vi "ROI entry-bundle parameter values.vi"(7 "XYZ_Coordinates":T1[](array[typedef]) {"Apparent Frame Size" format="%#_6f"; "Original FOV (um)" format="%#_6f"; "Pixels per miniscan" format="%#_6f"; "Dwell Time per pixel" format="%#_6f"; "Resolution" format="%#_6f"; "ROI group ID" format="%#_6f"; "Laser Power (%)" format="%#_6f"; "Zoom" format="%#_6f"; "Frame Size" format="%#_6f"; "Number of lines" format="%#_6f"; "Composite ID" format="%#_6f"; "Angle (deg)" format="%#_6f"; "ROI Time (ns)" format="%#_6f"; "ROI ID" format="%#_6f"; "Pixels in ROI" format="%#_6f"; "ROI index" format="%#_6f"; "Z stop" format="%#_6f"; "Y stop" format="%#_6f"; "X stop" format="%#_6f"; "Z start" format="%#_6f"; "X start" format="%#_6f"; "Y start" format="%#_6f"}, 8 "error in (no error)":errorcluster, 9 "Button Label.Text":string, 11 "Adj Timing for MC":bool) -> (0 "error out":errorcluster, 3 "AOL_Globals out":T2={"Imaging Protocol"=enum."AOL Z-Stack", "Number of POI"=0, "Number of Miniscans"=0, "Number of Trials"=0, "Number of Cycles "=0, "# Averaged Frames"=0, "Laser power (%)"=0, "Pockels (V)"=0.0, "Acquisition Length (sec)"=0.0, "Fill time (us)"=0.0, "POI Dwell time (us)"=0.0, "Miniscan Dwell time per pixel (us)"=0.0, "PMT 1"=0.0, "PMT 2"=0.0, "Back Apperture (mA)"=0.0, "Frame Size"=0, "Center Frequency"=0.0, "Field of View (um)"=175.0, "Field of View (norm)"=0.0, "DwellTime (us)"=0.0, "Ref Dwell Time (us)"=0.0, "Wavelength (nm)"=0.0, "Zoom"=0.0, "AOL Z"=0.0, "AOL Mode"=enum."Raster", "GridXY"=0.0, "GridZ"=0.0, "TriggerPeriod (sec)"=0.0, "Number of Pixels in Miniscan"=0, "Experiment folder path"=path "", "X centre"=0.0, "Y centre"=0.0, "Angle (degrees)"=0.0, "Angle Xs (degrees)"=0.0, "Angle Ys (degrees)"=0.0, "Plane Mode"=0, "Threshold"=[], "Regenerate Chirps"=FALSE, "Rectangle ROI length (pixels)"=0, "Rectangle ROI height (pixels)"=0, "AOD fill"=4900, "StartupDelay"=0, "Samples Wait after Trigger"=5080, "Slip Cycle"=600000, "Add Cycle"=TRUE, "Functional Mode"=enum."Point", "Z Start"=0.0, "Z Stop"=0.0, "# Planes"=0, "Total Pixels"=0, "Variable Miniscan Pixels"=[], "Use Variable Length"=FALSE, "Use Variable Resolution"=FALSE, "Laser power (%) at Z Start"=0, "Laser power (%) at Z Stop"=0, "Ref Z Step"=0} {"Angle Ys (degrees)" format="%#.6g"; "Angle Xs (degrees)" format="%#.6g"; "Plane Mode" items=["XY Plane", "XZ Plane", "YZ Plane", "arbitraryplane"]; "Frame Size" items=["100X100"=100, "128X128"=128, "200X200"=200, "256X256"=256, "512X512"=512, "1024x1024"=1024, "2048x2048"=2048]; "Back Apperture (mA)" format="%#.6g"; "Pockels (V)" format="%#.6g"; "PMT 2" format="%#.6g"; "PMT 1" format="%#.6g"; "Angle (degrees)" format="%#.6g"; "POI Dwell time (us)" format="%#.6g"})   [LabVIEW 2020]
uses:
  Typedefs/Controls/AOL_Globals.ctl
  Typedefs/Imaging Protocols enum.ctl
  Typedefs/Frame Size.ctl
  Typedefs/AOL modes.ctl
  Typedefs/Plane Mode.ctl
  Typedefs/Functional Mode.ctl
  Visualisation/Functional Imaging Viewer/Typedefs/ROI parameters data type.ctl
  <userlib>/_MGI/Application Control/MGI Change Detector/MGI Change Detector (T).vi
  Global Variables/General Globals.vi
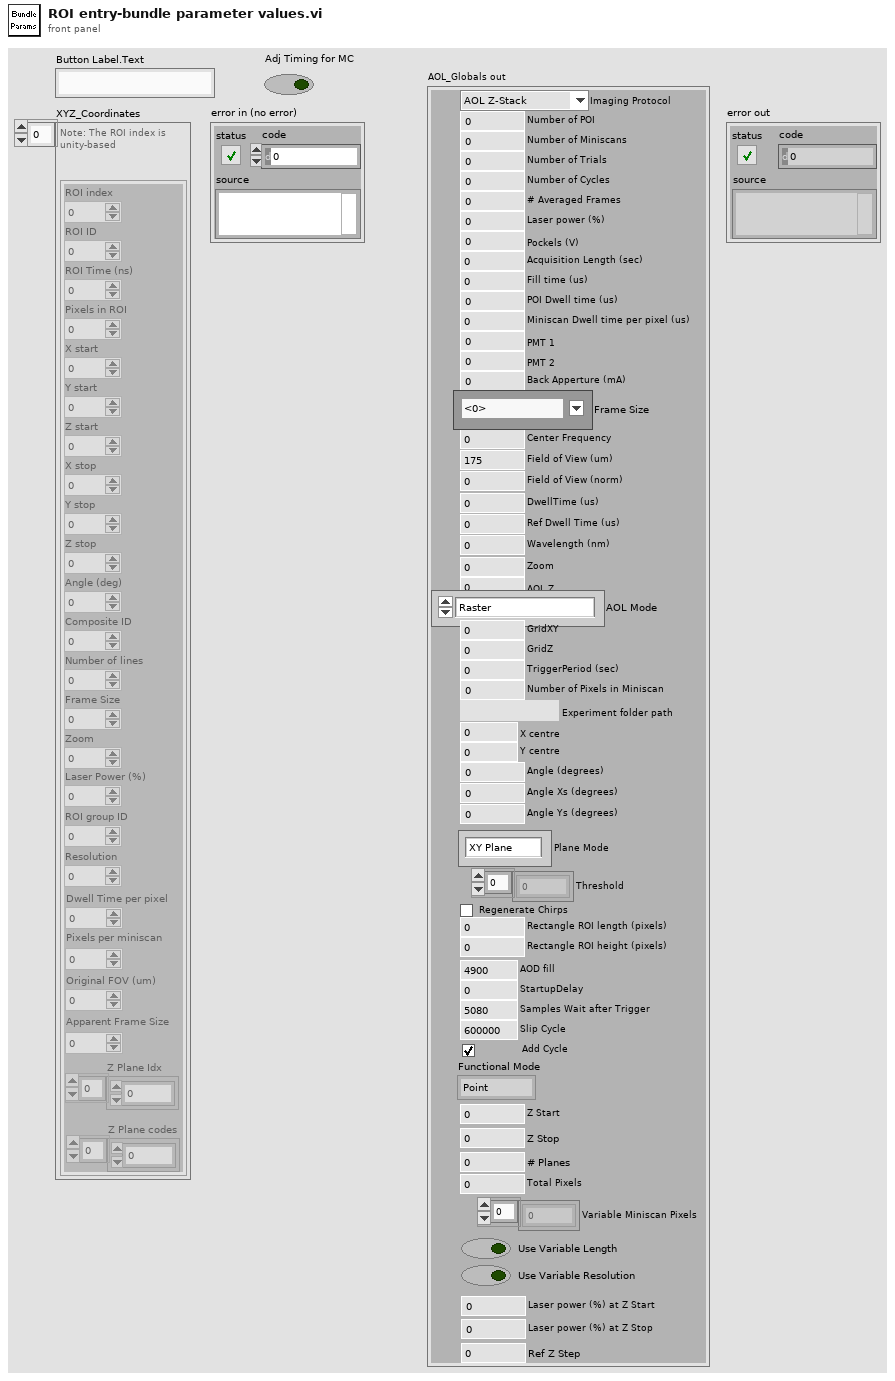
[diagram p1: front panel]
types:
  T1 = typedef "ROI parameters data type.ctl" = cluster{"ROI index":dbl, "ROI ID":dbl, "ROI Time (ns)":dbl, "Pixels in ROI":dbl, "X start":dbl, "Y start":dbl, "Z start":dbl, "X stop":dbl, "Y stop":dbl, "Z stop":dbl, "Angle (deg)":dbl, "Composite ID":dbl, "Number of lines":dbl, "Frame Size":dbl, "Zoom":dbl, "Laser Power (%)":dbl, "ROI group ID":dbl, "Resolution":dbl, "Dwell Time per pixel":dbl, "Pixels per miniscan":dbl, "Original FOV (um)":dbl, "Apparent Frame Size":dbl, "Z Plane Idx":i32[], "Z Plane codes":i32[]}
  T2 = typedef "AOL_Globals.ctl" = cluster{"Imaging Protocol":T3, "Number of POI":u16, "Number of Miniscans":u16, "Number of Trials":u16, "Number of Cycles ":u64, "# Averaged Frames":u16, "Laser power (%)":u8, "Pockels (V)":dbl, "Acquisition Length (sec)":dbl, "Fill time (us)":dbl, "POI Dwell time (us)":dbl, "Miniscan Dwell time per pixel (us)":dbl, "PMT 1":dbl, "PMT 2":dbl, "Back Apperture (mA)":dbl, "Frame Size":T4, "Center Frequency":dbl, "Field of View (um)":dbl, "Field of View (norm)":dbl, "DwellTime (us)":dbl, "Ref Dwell Time (us)":dbl, "Wavelength (nm)":dbl, "Zoom":dbl, "AOL Z":dbl, "AOL Mode":T5, "GridXY":dbl, "GridZ":dbl, "TriggerPeriod (sec)":dbl, "Number of Pixels in Miniscan":u16, "Experiment folder path":path, "X centre":dbl, "Y centre":dbl, "Angle (degrees)":dbl, "Angle Xs (degrees)":dbl, "Angle Ys (degrees)":dbl, "Plane Mode":T6, "Threshold":u16[], "Regenerate Chirps":bool, "Rectangle ROI length (pixels)":u16, "Rectangle ROI height (pixels)":u16, "AOD fill":u16, "StartupDelay":i32, "Samples Wait after Trigger":u16, "Slip Cycle":u32, "Add Cycle":bool, "Functional Mode":T7, "Z Start":dbl, "Z Stop":dbl, "# Planes":i32, "Total Pixels":i32, "Variable Miniscan Pixels":u16[], "Use Variable Length":bool, "Use Variable Resolution":bool, "Laser power (%) at Z Start":u8, "Laser power (%) at Z Stop":u8, "Ref Z Step":i8}
  T3 = typedef "Imaging Protocols enum.ctl" = enum16{"AOL Z-Stack", "Motor Z Stack", "Parameter Sweep", "Functional Acquisition", "Single Plane Acquisition", "Volume Acquisition", "Live Imaging", "Live Plane Imaging", "Live Volume Imaging"}
  T4 = typedef "Frame Size.ctl" = u16
  T5 = typedef "AOL modes.ctl" = enum16{"Raster", "Structural", "Pointing", "Mini Scan", "Alignment"}
  T6 = typedef "Plane Mode.ctl" = u16
  T7 = typedef "Functional Mode.ctl" = enum16{"Point", "Line", "Patch", "Plane", "Volume"}
  T8 = typedef "ROI ID Enum.ctl" = enum16{"Point", "MiniScan", "Comp. MiniScan", "Rectangle", "Comp. volume", "Arb. plane point", "None"}
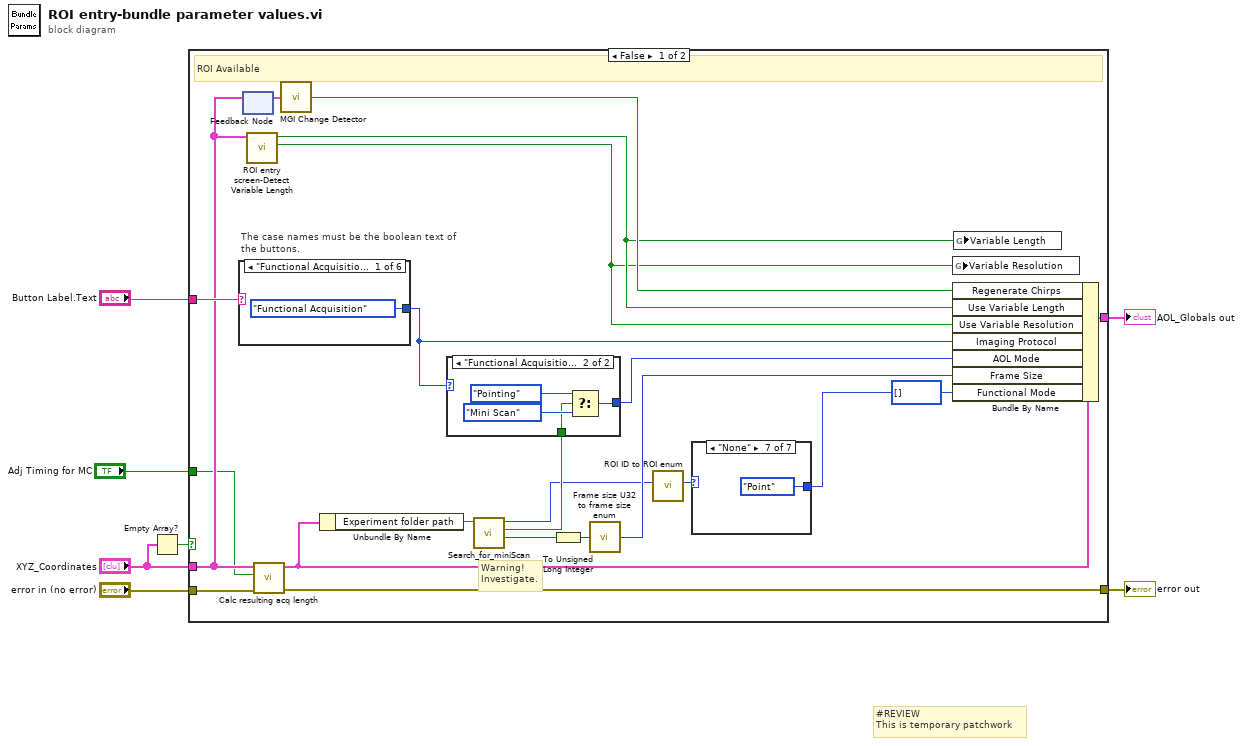
[diagram p0: block diagram]
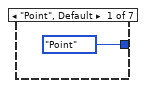
[diagram p2: hidden frame]
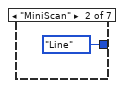
[diagram p3: hidden frame]
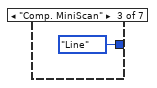
[diagram p4: hidden frame]
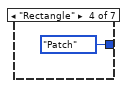
[diagram p5: hidden frame]
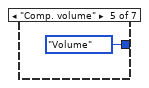
[diagram p6: hidden frame]
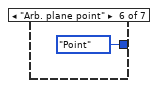
[diagram p7: hidden frame]
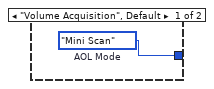
[diagram p8: hidden frame]
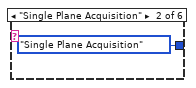
[diagram p9: hidden frame]
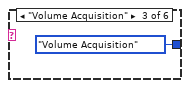
[diagram p10: hidden frame]
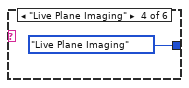
[diagram p11: hidden frame]
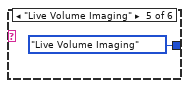
[diagram p12: hidden frame]
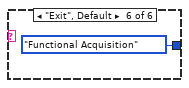
[diagram p13: hidden frame]
diagram:
  # "#REVIEW\nThis is temporary patchwork"
  n1 = Empty Array?(array="XYZ_Coordinates") -> (empty?=w5:bool)
  n2 = case shown="False" w5 {
    tunnel: "XYZ_Coordinates" -> [w12 _]
    tunnel: [w27 _] -> w7
    tunnel: [w26 _] -> w6
    tunnel: "Button Label.Text" -> [w24 _]
    tunnel: "error in (no error)" -> [w14 _]
    tunnel: "Adj Timing for MC" -> [w10 _]
    frame False {
      (unwired) u16[] [] ("Variable Miniscan Pixels")
      # "Warning!\nInvestigate."
      # "ROI Available"
      n3 = case "The case names must be the boolean text of the buttons." shown="\"Functional Acquisition\"" w24 {
        tunnel: [Imaging_Protocols_enum."Functional Acquisition" ("Imaging Protocol") Imaging_Protocols_enum."Single Plane Acquisition" ("Imaging Protocol") Imaging_Protocols_enum."Volume Acquisition" ("Imaging Protocol") Imaging_Protocols_enum."Live Plane Imaging" ("Imaging Protocol") Imaging_Protocols_enum."Live Volume Imaging" ("Imaging Protocol") Imaging_Protocols_enum."Functional Acquisition" ("Imaging Protocol")] -> w23
        frame "Functional Acquisition" {
        }
        frame "Single Plane Acquisition" {
        }
        frame "Volume Acquisition" {
        }
        frame "Live Plane Imaging" {
        }
        frame "Live Volume Imaging" {
        }
        frame "Exit", Default {
        }
      }
      n4 = feedback #1() -> (w28:T1[])  [unwired: 1 in]
      n5 = feedback-in #1(w12) -> ()
      n6 = call "ROI entry screen-Detect Variable Length.vi"("XYZ_Coordinates"=w12) -> ("VR ?"=w8:bool, "VL ?"=w9:bool)  [unwired: 8 in, 1 out]
      n7 = call "Calc resulting acq length.vi"("error in (no error)"=w14, "Adjust for MC ?"=w10, "XYZ_Coordinates"=w12) -> ("error out"=w27:errorcluster, "Output cluster"=w17:T2)  [unwired: 7 in]
      n8 = call-poly <userlib>:"MGI Change Detector.vi"("Value"=w28) -> ("Changed?"=w11:bool)
      n9 = Unbundle By Name(w17) -> ("Experiment folder path"=w25:path)
      n10 = call "Search_for_miniScan.vi"("AOL ZStack Path"=w25) -> ("Frame Size"=w20:i64, "POI/ROI"=w21:bool, "ROI ID"=w16:i64)  [unwired: 8 in]
      n11 = case shown="\"Functional Acquisition\"" w23 {
        tunnel: [w36 w39] -> w22
        tunnel: w21 -> [_ w38]
        frame "Volume Acquisition", Default {
          w36 = AOL_modes."Mini Scan"  # AOL Mode
        }
        frame "Functional Acquisition" {
          n12 = Select(t=AOL_modes."Pointing" ("AOL Mode"), s=w38, f=AOL_modes."Mini Scan" ("AOL Mode")) -> (s? t:f=w39:T5)
        }
      }
      n13 = To Unsigned Long Integer(number=w20) -> (unsigned 32bit integer=w19:u32)
      n14 = call "Frame size U32 to frame size enum.vi"("Frame Size U32"=w19) -> ("Value"=w18:T4)
      n15 = call "ROI ID to ROI enum.vi"("ROI ID"=w16) -> ("ROI Enum"=w15:T8)  [unwired: 6 in]
      n16 = case shown="\"None\"" w15 {
        tunnel: [Functional_Mode."Point" ("Functional Mode") Functional_Mode."Line" ("Functional Mode") Functional_Mode."Line" ("Functional Mode") Functional_Mode."Patch" ("Functional Mode") Functional_Mode."Volume" ("Functional Mode") Functional_Mode."Point" ("Functional Mode") Functional_Mode."Point" ("Functional Mode")] -> w13
        frame "Point", Default {
        }
        frame "MiniScan" {
        }
        frame "Comp. MiniScan" {
        }
        frame "Rectangle" {
        }
        frame "Comp. volume" {
        }
        frame "Arb. plane point" {
        }
        frame "None" {
        }
      }
      n17 = global write "General Globals.vi" "Variable Resolution"(w8) -> ()
      n18 = Bundle By Name(cluster=w17, "Regenerate Chirps"=w11, "Use Variable Length"=w9, "Use Variable Resolution"=w8, "Imaging Protocol"=w23, "AOL Mode"=w22, "Frame Size"=w18, "Functional Mode"=w13) -> (w26:T2)
      n19 = global write "General Globals.vi" "Variable Length"(w9) -> ()
    }
    frame True {
      # "No ROI Entered"
    }
  }
  "AOL_Globals out" <- w6
  "error out" <- w7
